vi "RejectionArea.vi"(4 "Prev Rej Area Data":bool, 5 "Current Rej Area Data":bool, 6 "No. Failure":refnum<vi>, 7 "No. Peg Rej":refnum<vi>, 9 "Rej Cntrl":refnum<vi>, 10 "No. Ring Rej":refnum<vi>, 11 "No. Success":refnum<vi>) -> (3 "Rejector Output":bool)   [LabVIEW 2016]
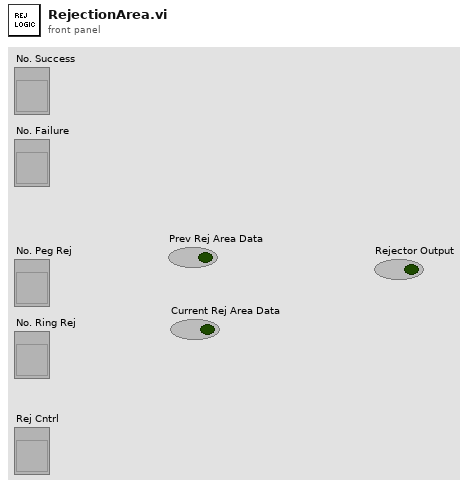
[diagram p1: front panel]
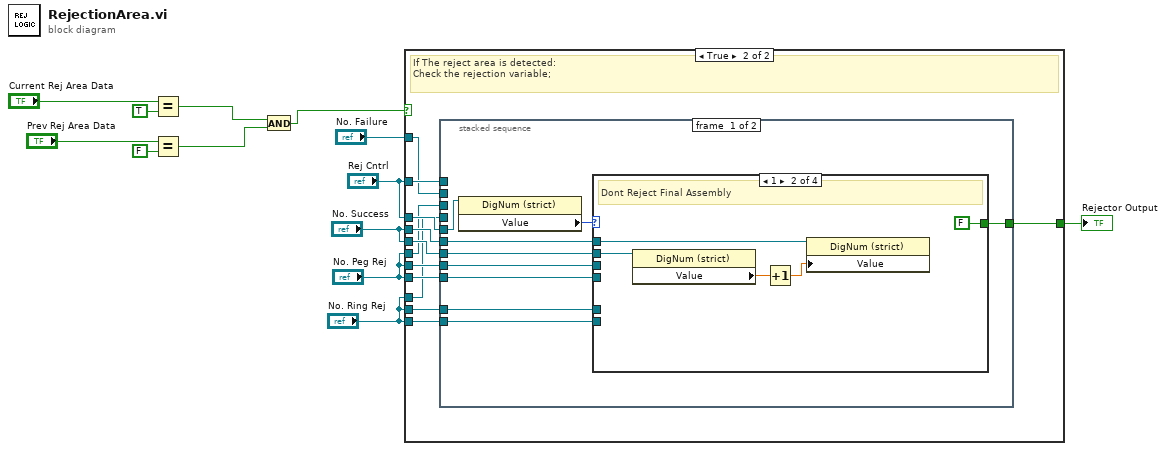
[diagram p0: block diagram]
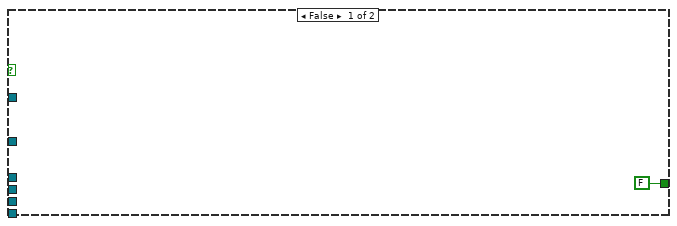
[diagram p2: hidden frame]
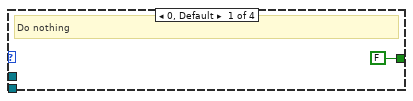
[diagram p3: hidden frame]
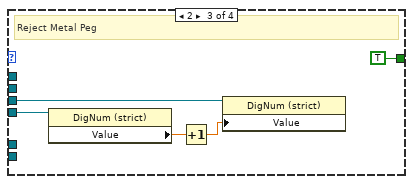
[diagram p4: hidden frame]
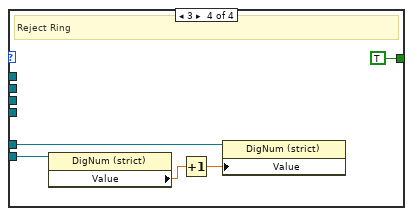
[diagram p5: hidden frame]
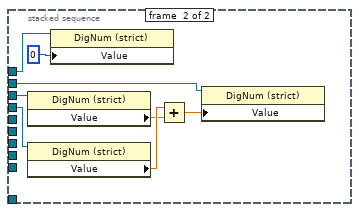
[diagram p6: hidden frame]
diagram:
  n1 = Equal?(x="Current Rej Area Data", y=TRUE) -> (x = y?=w2:bool)
  n2 = Equal?(x="Prev Rej Area Data", y=FALSE) -> (x = y?=w1:bool)
  n3 = And(x=w2, y=w1) -> (x .and. y?=w3:bool)
  n4 = case shown="True" w3 {
    tunnel: [FALSE w26] -> w13
    tunnel: "No. Success" -> [_ w25]
    tunnel: "No. Success" -> [_ w24]
    tunnel: "No. Peg Rej" -> [_ w23]
    tunnel: "No. Peg Rej" -> [_ w22]
    tunnel: "No. Ring Rej" -> [_ w21]
    tunnel: "No. Ring Rej" -> [_ w20]
    tunnel: "Rej Cntrl" -> [_ w19]
    tunnel: "Rej Cntrl" -> [_ w18]
    tunnel: "No. Peg Rej" -> [_ w17]
    tunnel: "No. Failure" -> [_ w16]
    tunnel: "No. Ring Rej" -> [_ w15]
    frame False {
    }
    frame True {
      # "If The reject area is detected:\nCheck the rejection variable;"
      n5 = stacked-sequence {
        tunnel: [w34 _] -> w26
        tunnel: w25 -> [w33 _]
        tunnel: w24 -> [w32 _]
        tunnel: w23 -> [w31 _]
        tunnel: w22 -> [w30 _]
        tunnel: w21 -> [w29 _]
        tunnel: w20 -> [w28 _]
        tunnel: w19 -> [w27 _]
        tunnel: w18 -> [_ w55]
        tunnel: w17 -> [_ w54]
        tunnel: w16 -> [_ w53]
        tunnel: w15 -> [_ w52]
        frame #0 {
          n6 = property class="DigNum (strict)"(reference=w27) -> ("Value"=w35:i8)  [unwired: 1 in, 2 out]
          n7 = case shown="1" w35 {
            tunnel: [FALSE FALSE TRUE TRUE] -> w34
            tunnel: w33 -> [_ w38 _ _]
            tunnel: w32 -> [_ w37 _ _]
            tunnel: w31 -> [_ _ w43 _]
            tunnel: w30 -> [_ _ w42 _]
            tunnel: w29 -> [_ _ _ w48]
            tunnel: w28 -> [_ _ _ w47]
            frame 0, Default {
              # "Do nothing"
            }
            frame 1 {
              # "Dont Reject Final Assembly"
              n8 = property class="DigNum (strict)"(reference=w38) -> ("Value"=w39:dbl)  [unwired: 1 in, 2 out]
              n9 = Increment(x=w39) -> (x+1=w40:dbl)
              n10 = property class="DigNum (strict)"(reference=w37, "Value"=w40) -> ()  [unwired: 1 in, 2 out]
            }
            frame 2 {
              # "Reject Metal Peg"
              n11 = property class="DigNum (strict)"(reference=w43) -> ("Value"=w44:dbl)  [unwired: 1 in, 2 out]
              n12 = Increment(x=w44) -> (x+1=w45:dbl)
              n13 = property class="DigNum (strict)"(reference=w42, "Value"=w45) -> ()  [unwired: 1 in, 2 out]
            }
            frame 3 {
              # "Reject Ring"
              n14 = property class="DigNum (strict)"(reference=w48) -> ("Value"=w50:dbl)  [unwired: 1 in, 2 out]
              n15 = Increment(x=w50) -> (x+1=w49:dbl)
              n16 = property class="DigNum (strict)"(reference=w47, "Value"=w49) -> ()  [unwired: 1 in, 2 out]
            }
          }
        }
        frame #1 {
          n17 = property class="DigNum (strict)"(reference=w54) -> ("Value"=w57:dbl)  [unwired: 1 in, 2 out]
          n18 = property class="DigNum (strict)"(reference=w52) -> ("Value"=w58:dbl)  [unwired: 1 in, 2 out]
          n19 = property class="DigNum (strict)"(reference=w55, "Value"=i8 0 ("Rejection Control")) -> ()  [unwired: 1 in, 2 out]
          n20 = Add(x=w58, y=w57) -> (x+y=w56:dbl)
          n21 = property class="DigNum (strict)"(reference=w53, "Value"=w56) -> ()  [unwired: 1 in, 2 out]
        }
      }
    }
  }
  "Rejector Output" <- w13
